vi "Error Monitor Subpanel.vi"(11 "CIF_UI in":refnum<class "CIF_UI.lvclass">) -> ()   [LabVIEW 2021, in "CIF Manager UI.lvlib"]
uses:
  CIF Manager UI.lvlib
  CIFUI/CIF_UI.lvclass
  CIFUI/Typedef/Core UI References.ctl
  CIFUI/CIF_UI.lvclass/CIF_UI.ctl
  CIFPluginManager/gRPC/CIF_Manager_client/RPC Messages/cif_manager_OrchConfig.ctl
  CIFPluginManager/gRPC/CIF_Manager_client/RPC Messages/cif_manager_OrchestrationLanguage.ctl
  CIFUI/UI Element Update/Empty Tree.vi
  CIFUI/UI Element Update/Empty Table.vi
  CIFUI/UI Element Update/Initialize Manager Tab.vi
  CIFPluginManager/gRPC/CIF_Manager_Client_Wrapper/CIFManagerClientWrapper.lvlib
  CIFPluginManager/gRPC/CIF_Manager_client/CIF_Manager_client.lvlib
panel:
  in  "Plugin Status":string[][](table)
  out "Orchestration":string
  in  "Generate Orchestration":bool
  in  "Errors 2":i32(listbox)=-1
  in  "Reset Errors":bool
  out "Config":string
  in  "Get Config":bool
  in  "Reset Config":bool
  in  "Get All Errors":bool
  in  "All Config":bool
  in  "File Name":string="orchestrate.py"
  in  "Start Timestamp":u64
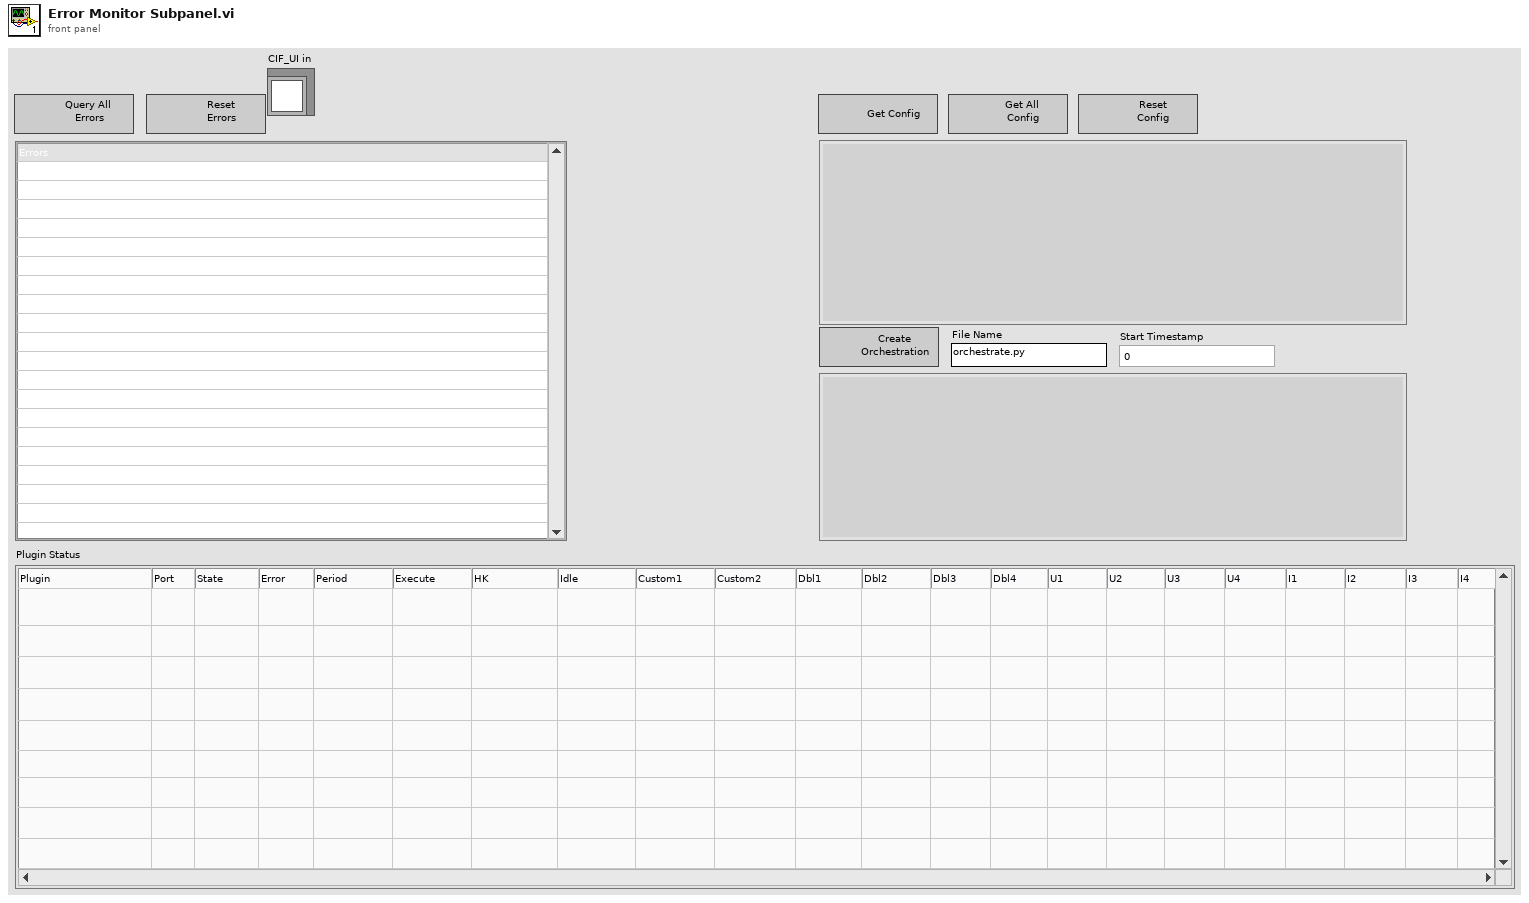
[diagram p1: front panel]
types:
  T1 = typedef "CIF_UI.lvclass/Core UI References.ctl" = cluster{"Discovered Plugins":refnum<vi>, "Discovered Plugins Valid":bool, "Loaded Plugins":refnum<vi>, "Loaded Plugins Valid":bool, "Publisher Channels":refnum<vi>, "Publisher Channels Valid":bool, "Subscriber Channels":refnum<vi>, "Subscriber Channels Valid":bool, "Plugin Status":refnum<vi>, "Plugin Status Valid":bool, "Channel Connection":refnum<vi>, "Channel Connection Valid":bool, "New Plugin Load":refnum<vi>, "New Plugin Load Valid":bool, "Errors":refnum<vi>, "Errors Valid":bool, "Plugin to Abort":refnum<vi>, "Plugin to Abort Valid":bool, "Connection":refnum<vi>, "Connection Valid":bool, "Exit":refnum<vi>, "Exit Valid":bool, "Run Listen":refnum<vi>, "Run Listen Valid":bool, "CIF Manager Tab":refnum<vi>, "Manger Tab Valid":bool, "Clear Local Error":refnum<vi>, "Clear Local Error Valid":bool, "Local Error":refnum<vi>, "Local Error Valid":bool, "System Errors":refnum<vi>, "System Errors Valid":bool}
  T2 = typedef "CIF_Manager_client.lvlib/cif_manager_OrchConfig.ctl" = cluster{"start_timestamp":u64, "create_file":bool, "orchestration_language":T3, "filename":string, "default_ip":string}
  T3 = typedef "CIF_Manager_client.lvlib/cif_manager_OrchestrationLanguage.ctl" = enum32{"NULL", "PYTHON"}
  T4 = typedef "grpc-lvsupport-release.lvlib/grpcId.ctl" = u64
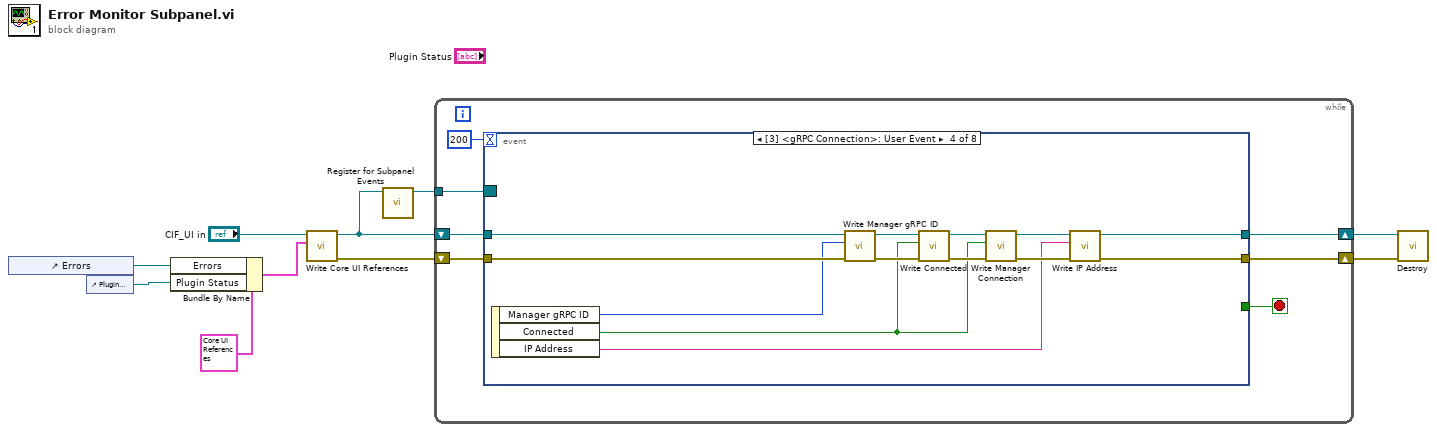
[diagram p0: block diagram]
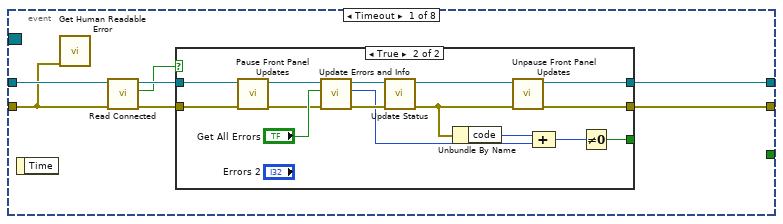
[diagram p2: hidden frame]
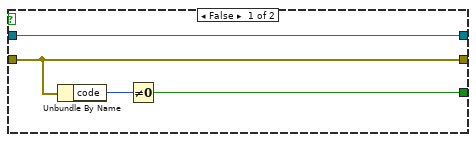
[diagram p3: hidden frame]
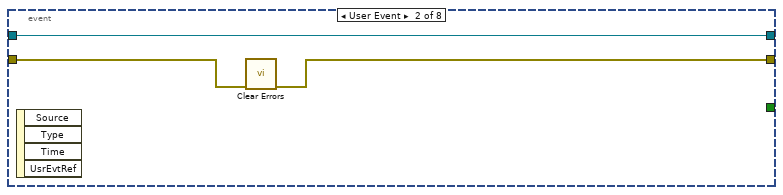
[diagram p4: hidden frame]
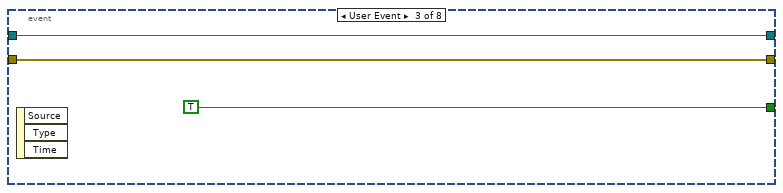
[diagram p5: hidden frame]
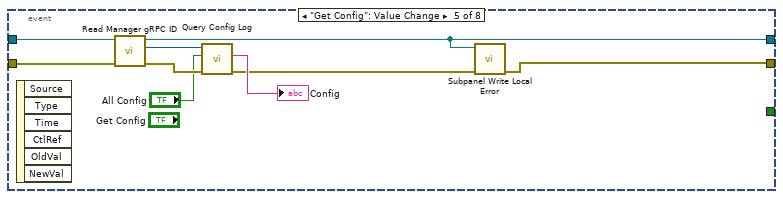
[diagram p6: hidden frame]
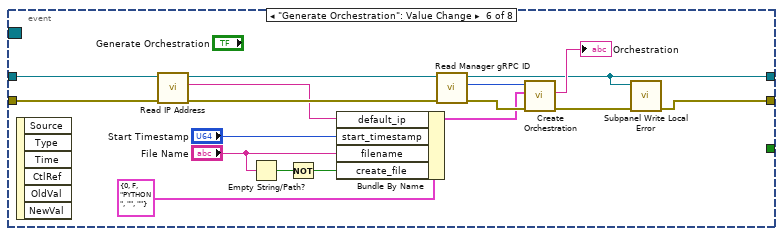
[diagram p7: hidden frame]
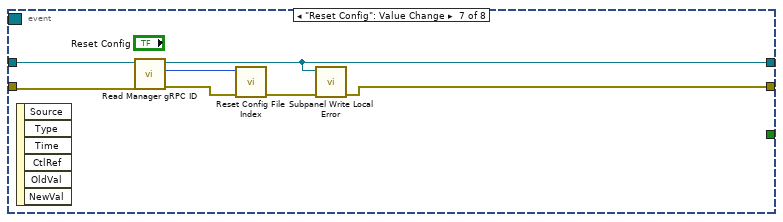
[diagram p8: hidden frame]
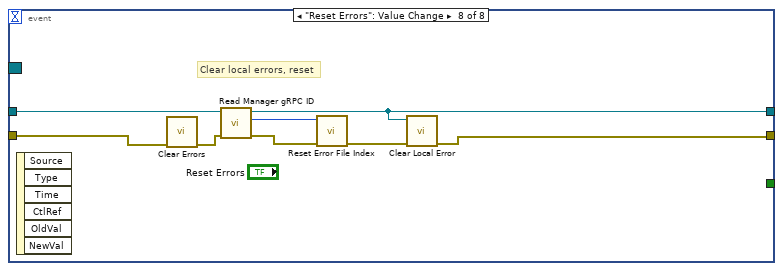
[diagram p9: hidden frame]
diagram:
  n1 = control-ref of="Errors"() -> (w8:refnum<vi>)
  n2 = control-ref of="Plugin Status"() -> (w4:refnum<vi>)
  n3 = Bundle By Name(cluster=T1 {"Discovered Plugins"=refnum, "Discovered Plugins Valid"=FALSE, "Loaded Plugins"=refnum, "Loaded Plugins Valid"=FALSE, "Publisher Channels"=refnum, "Publisher Channels Valid"=FALSE, "Subscriber Channels"=refnum, "Subscriber Channels Valid"=FALSE, "Plugin Status"=refnum, "Plugin Status Valid"=FALSE, "Channel Connection"=refnum, "Channel Connection Valid"=FALSE, "New Plugin Load"=refnum, "New Plugin Load Valid"=FALSE, "Errors"=refnum, "Errors Valid"=FALSE, "Plugin to Abort"=refnum, "Plugin to Abort Valid"=FALSE, "Connection"=refnum, "Connection Valid"=FALSE, "Exit"=refnum, "Exit Valid"=FALSE, "Run Listen"=refnum, "Run Listen Valid"=FALSE, "CIF Manager Tab"=refnum, "Manger Tab Valid"=FALSE, "Clear Local Error"=refnum, "Clear Local Error Valid"=FALSE, "Local Error"=refnum, "Local Error Valid"=FALSE, "System Errors"=refnum, "System Errors Valid"=FALSE} ("UI References"), "Errors"=w8, "Plugin Status"=w4) -> (w5:T1)
  n4 = call "Write Core UI References.vi"("UI References"=w5, "CIF_UI in"="CIF_UI in") -> ("error out"=w6:errorcluster, "CIF_UI out"=w2:refnum<class "CIF_UI.lvclass">)  [unwired: 8 in]
  n5 = call "Register for Subpanel Events.vi"("CIF_UI in"=w2) -> ("Event Registration Refnum"=w1:refnum<event-registration>)  [unwired: 9 in, 1 out]
  n6 = while {
    shift-right: [w12] -> w9
    shift-left: w2 -> [w15]
    shift-right: [w13] -> w10
    shift-left: w6 -> [w14]
    tunnel: w1 -> [w11]
    stop <- w16 stop-if-true
    n7 = event shown="[3] <gRPC Connection>: User Event" {
      selector: w11 -> [_ _ _ _ _ _ _ _]
      dyn-events: _ -> [_ _ _ _ _ _ _ _]
      timeout: 200 -> [_ _ _ _ _ _ _ _]
      tunnel: [_ _ TRUE _ _ _ _ _] -> w16
      tunnel: w15 -> [w19 w44 w48 w56 w67 w85 w93 w101]
      tunnel: w14 -> [w18 w46 w47 w55 w66 w84 w92 w100]
      tunnel: [w21 w45 w47 w53 w63 w72 w89 w96] -> w13
      tunnel: [w24 w44 w48 w54 w65 w74 w91 w97] -> w12
      event Timeout {
        n8 = event-data() -> ()  [unwired: 1 in, 1 out]
        n9 = call "Get Human Readable Error.vi"("error in (no error)"=w18) -> ()  [unwired: 10 in, 1 out]
        n10 = call "Read Connected.vi"("error in (no error)"=w18, "CIF_UI in"=w19) -> ("error out"=w22:errorcluster, "Connected"=w20:bool, "CIF_UI out"=w23:refnum<class "CIF_UI.lvclass">)  [unwired: 7 in]
        n11 = case shown="True" w20 {
          tunnel: w22 -> [w27 w31]
          tunnel: [w27 w34] -> w21
          tunnel: w23 -> [w28 w32]
          tunnel: [w28 w33] -> w24
          tunnel: [w25 w41] -> _
          frame False {
            n12 = Unbundle By Name(w27) -> ("code"=w26:i32)
            n13 = Not Equal To 0?(x=w26) -> (x != 0?=w25:bool)
          }
          frame True {
            n14 = call "Pause Front Panel Updates.vi"("error in (no error)"=w31, "CIF_UI in"=w32) -> ("error out"=w29:errorcluster, "CIF_UI out"=w30:refnum<class "CIF_UI.lvclass">)  [unwired: 8 in]
            n15 = call "Update Errors and Info.vi"("error in (no error)"=w29, "Get All Errors"="Get All Errors", "CIF_UI in"=w30) -> ("error out"=w40:errorcluster, "Error Count"=w37:i32, "CIF_UI out"=w39:refnum<class "CIF_UI.lvclass">)  [unwired: 5 in, 1 out]
            n16 = call "Update Status.vi"("error in (no error)"=w40, "CIF_UI in"=w39) -> ("error out"=w35:errorcluster, "CIF_UI out"=w36:refnum<class "CIF_UI.lvclass">)  [unwired: 8 in]
            n17 = Unbundle By Name(w35) -> ("code"=w43:i32)
            n18 = call "Unpause Front Panel Updates.vi"("error in (no error)"=w35, "CIF_UI in"=w36) -> ("error out"=w34:errorcluster, "CIF_UI out"=w33:refnum<class "CIF_UI.lvclass">)  [unwired: 8 in]
            n19 = Compound Arithmetic op=ADD(w43, w37) -> (w42:i32)
            n20 = Not Equal To 0?(x=w42) -> (x != 0?=w41:bool)
          }
        }
      }
      event User Event {
        n21 = event-data() -> ()  [unwired: 1 in, 4 out]
        n22 = call <vilib>:"Clear Errors.vi"("error in (no error)"=w46) -> ("error out"=w45:errorcluster)  [unwired: 5 in, 1 out]
      }
      event User Event {
        n23 = event-data() -> ()  [unwired: 1 in, 3 out]
      }
      event User Event {
        n24 = event-data() -> ("Manager gRPC ID"=w50:T4, "Connected"=w51:bool, "IP Address"=w52:string)  [unwired: 1 in]
        n25 = call "Write Manager gRPC ID.vi"("error in (no error)"=w55, "gRPCid"=w50, "CIF_UI in"=w56) -> ("error out"=w61:errorcluster, "CIF_UI out"=w62:refnum<class "CIF_UI.lvclass">)  [unwired: 7 in]
        n26 = call "Write Connected.vi"("error in (no error)"=w61, "Connected"=w51, "CIF_UI in"=w62) -> ("error out"=w59:errorcluster, "CIF_UI out"=w60:refnum<class "CIF_UI.lvclass">)  [unwired: 7 in]
        n27 = call "Write Manager Connection.vi"("error in (no error)"=w59, "Manager Connection"=w51, "CIF_UI in"=w60) -> ("error out"=w57:errorcluster, "CIF_UI out"=w58:refnum<class "CIF_UI.lvclass">)  [unwired: 7 in]
        n28 = call "Write IP Address.vi"("error in (no error)"=w57, "IP Address"=w52, "CIF_UI in"=w58) -> ("error out"=w53:errorcluster, "CIF_UI out"=w54:refnum<class "CIF_UI.lvclass">)  [unwired: 7 in]
      }
      event "Get Config": Value Change {
        n29 = event-data() -> ()  [unwired: 1 in, 6 out]
        n30 = call "Read Manager gRPC ID.vi"("error in (no error)"=w66, "CIF_UI in"=w67) -> ("error out"=w70:errorcluster, "Manager gRPCid"=w71:T4, "CIF_UI out"=w65:refnum<class "CIF_UI.lvclass">)  [unwired: 7 in]
        n31 = call "Query Config Log.vi"("error in"=w70, "query_all"="All Config", "gRPC ID in"=w71) -> ("error out"=w64:errorcluster, "Config"=→"Config":string)  [unwired: 6 in, 1 out]
        n32 = call "Subpanel Write Local Error.vi"("error in (no error)"=w64, "CIF_UI in"=w65) -> ("error out"=w63:errorcluster)  [unwired: 9 in]
      }
      event "Generate Orchestration": Value Change {
        n33 = event-data() -> ()  [unwired: 1 in, 6 out]
        n34 = call "Read IP Address.vi"("error in (no error)"=w84, "CIF_UI in"=w85) -> ("error out"=w82:errorcluster, "IP address"=w79:string, "CIF_UI out"=w83:refnum<class "CIF_UI.lvclass">)  [unwired: 7 in]
        n35 = Empty String/Path?(string/path="File Name") -> (empty?=w77:bool)
        n36 = Not(x=w77) -> (.not. x?=w76:bool)
        n37 = Bundle By Name(cluster=T2 {"start_timestamp"=0, "create_file"=FALSE, "orchestration_language"=enum."PYTHON", "filename"="", "default_ip"=""} ("Orchestration Config"), "default_ip"=w79, "start_timestamp"="Start Timestamp", "filename"="File Name", "create_file"=w76) -> (w80:T2)
        n38 = call "Read Manager gRPC ID.vi"("error in (no error)"=w82, "CIF_UI in"=w83) -> ("error out"=w86:errorcluster, "Manager gRPCid"=w88:T4, "CIF_UI out"=w74:refnum<class "CIF_UI.lvclass">)  [unwired: 7 in]
        n39 = call "Create Orchestration.vi"("error in"=w86, "Orchestration Config"=w80, "gRPC ID in"=w88) -> ("error out"=w73:errorcluster, "Orchestration Script"=→"Orchestration":string)  [unwired: 6 in, 1 out]
        n40 = call "Subpanel Write Local Error.vi"("error in (no error)"=w73, "CIF_UI in"=w74) -> ("error out"=w72:errorcluster)  [unwired: 9 in]
      }
      event "Reset Config": Value Change {
        n41 = event-data() -> ()  [unwired: 1 in, 6 out]
        n42 = call "Read Manager gRPC ID.vi"("error in (no error)"=w92, "CIF_UI in"=w93) -> ("error out"=w94:errorcluster, "Manager gRPCid"=w95:T4, "CIF_UI out"=w91:refnum<class "CIF_UI.lvclass">)  [unwired: 7 in]
        n43 = call "Reset Config File Index.vi"("error in"=w94, "gRPC ID in"=w95) -> ("error out"=w90:errorcluster)  [unwired: 8 in, 1 out]
        n44 = call "Subpanel Write Local Error.vi"("error in (no error)"=w90, "CIF_UI in"=w91) -> ("error out"=w89:errorcluster)  [unwired: 9 in]
      }
      event "Reset Errors": Value Change {
        # "Clear local errors, reset"
        n45 = event-data() -> ()  [unwired: 1 in, 6 out]
        n46 = call <vilib>:"Clear Errors.vi"("error in (no error)"=w100) -> ("error out"=w99:errorcluster)  [unwired: 5 in, 1 out]
        n47 = call "Read Manager gRPC ID.vi"("error in (no error)"=w99, "CIF_UI in"=w101) -> ("error out"=w102:errorcluster, "Manager gRPCid"=w103:T4, "CIF_UI out"=w97:refnum<class "CIF_UI.lvclass">)  [unwired: 7 in]
        n48 = call "Reset Error File Index.vi"("error in"=w102, "gRPC ID in"=w103) -> ("error out"=w98:errorcluster)  [unwired: 8 in, 1 out]
        n49 = call "Clear Local Error.vi"("error in (no error)"=w98, "CIF_UI in"=w97) -> ("error out"=w96:errorcluster)  [unwired: 9 in]
      }
    }
  }
  n50 = call "Destroy.vi"("error in (no error)"=w10, "CIF_UI in"=w9) -> ()  [unwired: 8 in, 2 out]
